vi "User Permissions Number to Cluster.vi"(1 "User Permissions":i32) -> (0 "User Permisions":T1)   [LabVIEW 2011]
uses:
  User Permissions.ctl
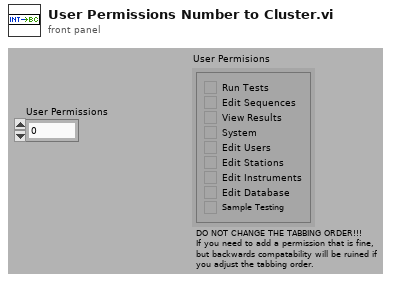
[diagram p1: front panel]
types:
  T1 = typedef "User Permissions.ctl" = cluster{"Run Tests":bool, "Edit Sequences":bool, "View Results":bool, "System":bool, "Edit Users":bool, "Edit Stations":bool, "Edit Instruments":bool, "Edit Database":bool, "Sample Testing":bool}
  T2 = cluster{"Boolean array[0]":bool, "Boolean array[1]":bool, "Boolean array[2]":bool, "Boolean array[3]":bool, "Boolean array[4]":bool, "Boolean array[5]":bool, "Boolean array[6]":bool, "Boolean array[7]":bool, "Boolean array[8]":bool}
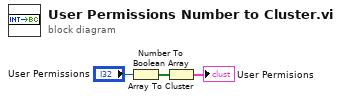
[diagram p0: block diagram]
diagram:
  n1 = Number To Boolean Array(number="User Permissions") -> (Boolean array=w1:bool[])
  n2 = Array To Cluster(array=w1) -> (cluster=→"User Permisions":T2)
